vi "get device count.vi"(8 "error in (no error)":errorcluster) -> (0 "error out":errorcluster, 3 "Device Count":u32)   [LabVIEW 2015, in "rtlsdr.lvlib"]
doc: "Gets the number of RTLSDR devices detected in the system."
uses:
  rtlsdr.lvlib
  rtlsdr/rtlsdr.dll
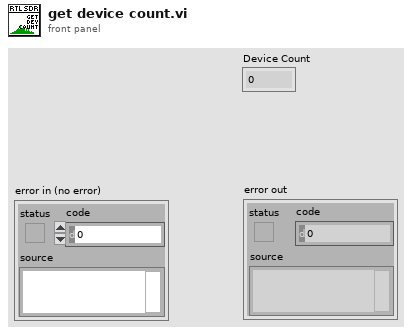
[diagram p1: front panel]
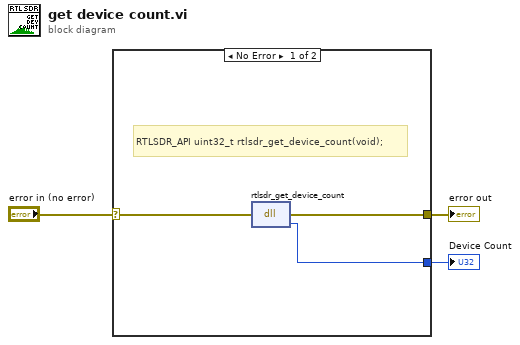
[diagram p0: block diagram]
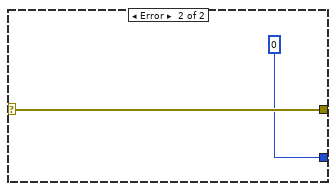
[diagram p2: hidden frame]
diagram:
  n1 = case shown="No Error" "error in (no error)" {
    selector: "error in (no error)" -> [w6 w8]
    tunnel: [w4 w8] -> w3
    tunnel: [w5 u32 0 ("return type")] -> w1
    frame No Error {
      # "RTLSDR_API uint32_t rtlsdr_get_device_count(void);"
      n2 = dll-call lib="C:/Users/TheDoctor/Documents/Projects/Labview Libraries/rtlsdr/rtlsdr.*" fn="rtlsdr_get_device_count"(error in=w6) -> (error out=w4:errorcluster, "return type"=w5:u32)  [unwired: 2 in, 1 out]
    }
    frame Error {
    }
  }
  "error out" <- w3
  "Device Count" <- w1
